vi "Spectrometer Triax 550 (N.O.).vi"(7 "Force Reset? (F)":bool, 8 "error in (no error)":errorcluster, 9 "VISA Resource Name":refnum<visa-resource-name>="GPIB0::1::INSTR", 10 "Ref to a Status Box":refnum<vi>, 11 "Cluster In":T4) -> (0 "error out":errorcluster, 3 "Cluster Out":T4)   [LabVIEW 2012]
uses:
  JY-SPEX-TRIAX/controls.llb/Monochromator System Number.ctl
  JY-SPEX-TRIAX/controls.llb/Mirror Position.ctl
  JY-SPEX-TRIAX/controls.llb/Turret Position (TRIAX).ctl
  JY-SPEX-TRIAX/JY-SPEX-TRIAX.lvlib
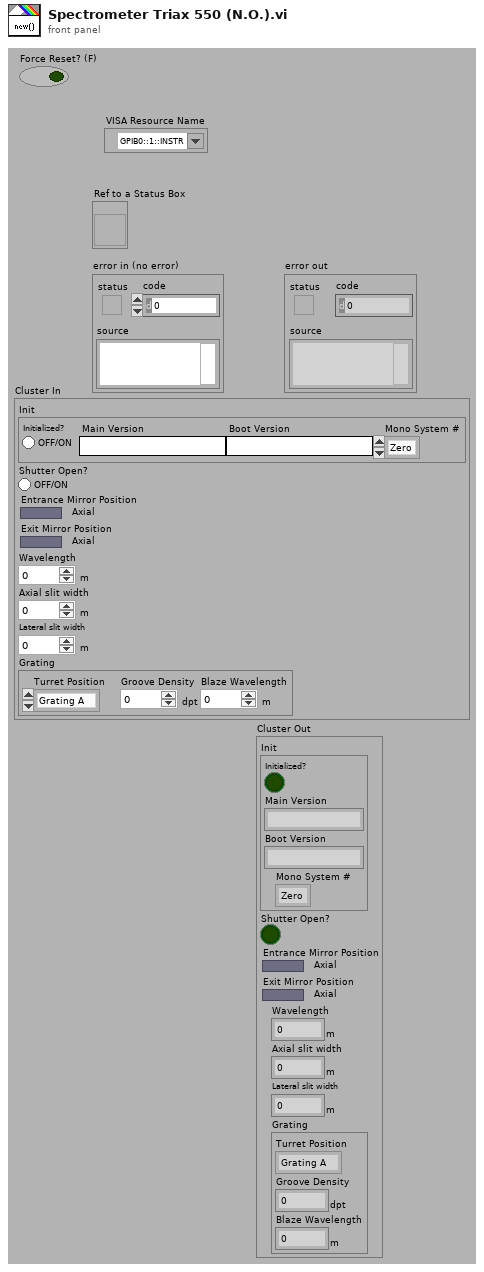
[diagram p1: front panel]
types:
  T1 = typedef "JY-SPEX-TRIAX.lvlib/Monochromator System Number.ctl" = enum16{"Zero", "One"}
  T2 = typedef "JY-SPEX-TRIAX.lvlib/Mirror Position.ctl" = bool
  T3 = typedef "JY-SPEX-TRIAX.lvlib/Turret Position (TRIAX).ctl" = enum16{"Grating A", "Grating B", "Grating C"}
  T4 = cluster{"Init":cluster{"Initialized?":bool, "Main Version":string, "Boot Version":string, "Mono System #":T1}, "Shutter Open?":bool, "Entrance Mirror Position":T2, "Exit Mirror Position":T2, "Wavelength":dbl[unit], "Axial slit width":dbl[unit], "Lateral slit width":dbl[unit], "Grating":cluster{"Turret Position":T3, "Groove Density":dbl[unit], "Blaze Wavelength":dbl[unit]}}
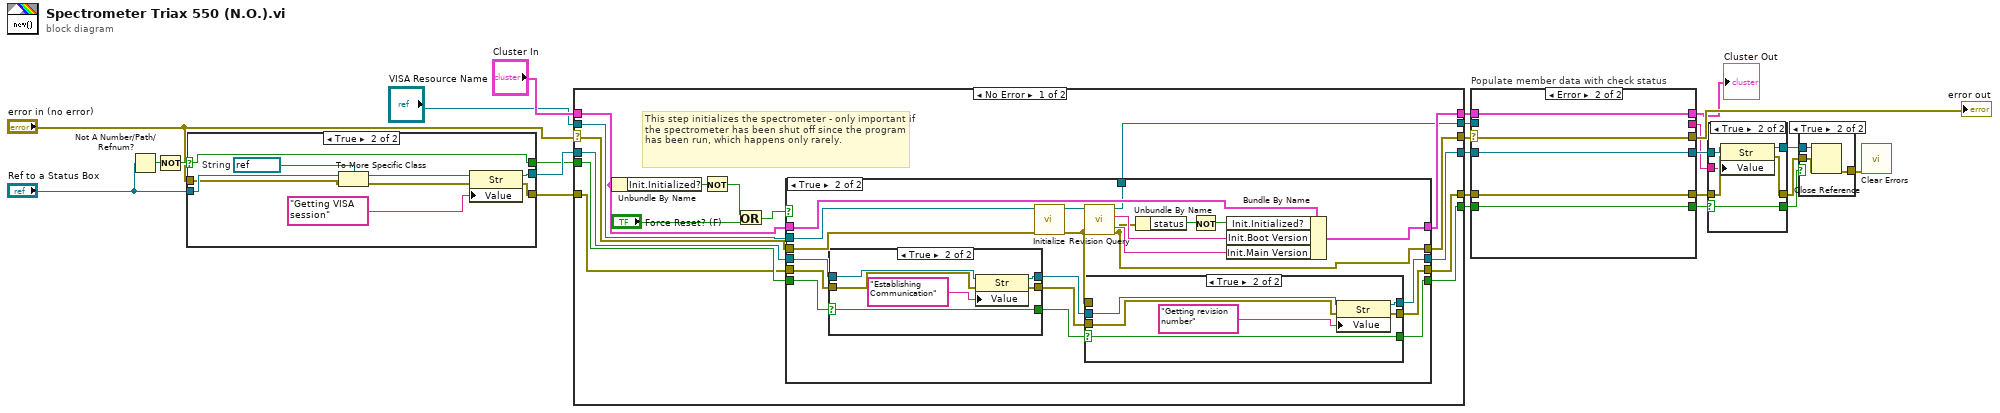
[diagram p0: block diagram]
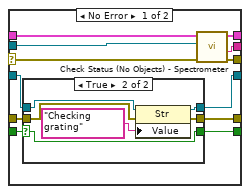
[diagram p2: hidden frame]
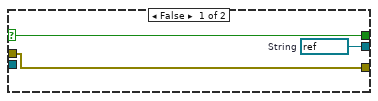
[diagram p4: hidden frame]
diagram:
  n1 = Not A Number/Path/Refnum?(number/path/refnum="Ref to a Status Box") -> (NaN/Path/Refnum?=w19:bool)
  n2 = Not(x=w19) -> (.not. x?=w7:bool)
  n3 = case shown="True" w7 {
    selector: w7 -> [w27 w34]
    tunnel: "error in (no error)" -> [w28 w29]
    tunnel: [w28 w37] -> w23
    tunnel: "Ref to a Status Box" -> [_ w32]
    tunnel: [w26 w35] -> w25
    tunnel: [w27 w34] -> w24
    frame False {
      w26 = refnum<vi> refnum  # String
    }
    frame True {
      w33 = refnum<vi> refnum  # String
      n4 = To More Specific Class(target class=w33, reference=w32, error in=w29) -> (specific class reference=w30:refnum<vi>, error out=w31:errorcluster)
      n5 = property class="Str"(reference=w30, error in=w31, "Value"="Getting VISA session") -> (reference out=w35:refnum<vi>, error out=w37:errorcluster)
    }
  }
  n6 = case shown="No Error" "error in (no error)" {
    selector: "error in (no error)" -> [w44 w104]
    tunnel: [w47 w104] -> w6
    tunnel: "Cluster In" -> [w43 w103]
    tunnel: "VISA Resource Name" -> [w53 w99]
    tunnel: [w52 w103] -> w18
    tunnel: w25 -> [w51 w102]
    tunnel: [w48 w102] -> w16
    tunnel: w24 -> [w50 w101]
    tunnel: [w49 w101] -> w14
    tunnel: w23 -> [w46 w100]
    tunnel: [w45 w100] -> w11
    tunnel: [w38 w99] -> w1
    frame No Error {
      # "This step initializes the spectrometer - only important if the spectrometer has been shut off since the program has been run, which happens only rarely."
      n7 = Unbundle By Name(w43) -> ("Init.Initialized?"=w41:bool)
      n8 = Not(x=w41) -> (.not. x?=w42:bool)
      n9 = Or(x=w42, y="Force Reset? (F)") -> (x .or. y?=w39:bool)
      n10 = case shown="True" w39 {
        tunnel: w43 -> [w59 w76]
        tunnel: w53 -> [w54 w75]
        tunnel: [w59 w62] -> w52
        tunnel: w51 -> [w57 w74]
        tunnel: w50 -> [w55 w73]
        tunnel: [w55 w71] -> w49
        tunnel: [w57 w69] -> w48
        tunnel: [w58 w61] -> w47
        tunnel: w46 -> [w56 w68]
        tunnel: [w56 w66] -> w45
        tunnel: w44 -> [w58 w65]
        tunnel: [w54 w60] -> w38
        frame False {
        }
        frame True {
          n11 = case shown="True" w73 {
            selector: w73 -> [w90 w93]
            tunnel: w68 -> [w91 w98]
            tunnel: [w91 w97] -> w67
            tunnel: w74 -> [w92 w96]
            tunnel: [w92 w94] -> w70
            tunnel: [w90 w93] -> w72
            frame False {
            }
            frame True {
              n12 = property class="Str"(reference=w96, error in=w98, "Value"="Establishing Communication") -> (reference out=w94:refnum<vi>, error out=w97:errorcluster)
            }
          }
          n13 = call "Initialize.vi"("error in (no error)"=w65, "VISA resource name"=w75) -> ("error out"=w63:errorcluster, "VISA resource name out"=w80:refnum<visa-resource-name>)  [unwired: 8 out]
          n14 = call "Revision Query.vi"("error in (no error)"=w63, "VISA resource name"=w80) -> ("error out"=w61:errorcluster, "Main Firmware Revision"=w77:string, "Boot Firmware Revision"=w78:string, "VISA resource name out"=w60:refnum<visa-resource-name>)  [unwired: 6 out]
          n15 = case shown="True" w72 {
            selector: w72 -> [w81 w84]
            tunnel: w67 -> [w82 w89]
            tunnel: [w82 w88] -> w66
            tunnel: w70 -> [w83 w87]
            tunnel: [w83 w85] -> w69
            tunnel: [w81 w84] -> w71
            tunnel: w63 -> [_ _]
            frame False {
            }
            frame True {
              n16 = property class="Str"(reference=w87, error in=w89, "Value"="Getting revision number") -> (reference out=w85:refnum<vi>, error out=w88:errorcluster)
            }
          }
          n17 = Unbundle By Name(w61) -> ("status"=w79:bool)
          n18 = Not(x=w79) -> (.not. x?=w64:bool)
          n19 = Bundle By Name(cluster=w76, "Init.Initialized?"=w64, "Init.Boot Version"=w78, "Init.Main Version"=w77) -> (w62:T4)
        }
      }
    }
    frame Error {
    }
  }
  n20 = case "Populate member data with check status" shown="Error" w6 {
    selector: w6 -> [w107 w129]
    tunnel: w18 -> [w106 w130]
    tunnel: [w116 w129] -> w17
    tunnel: [w115 w130] -> w3
    tunnel: w16 -> [w114 w127]
    tunnel: [w113 w127] -> w15
    tunnel: w14 -> [w112 w128]
    tunnel: [w111 w128] -> w13
    tunnel: [w110 w126] -> w12
    tunnel: w11 -> [w109 w126]
    tunnel: [w108 _] -> w10
    tunnel: w1 -> [w105 _]
    frame No Error {
      n21 = case shown="True" w112 {
        selector: w112 -> [w119 w123]
        tunnel: [w117 w125] -> w110
        tunnel: [w119 w123] -> w111
        tunnel: [w118 w122] -> w113
        tunnel: w109 -> [w117 w121]
        tunnel: w114 -> [w118 w120]
        frame False {
        }
        frame True {
          n22 = property class="Str"(reference=w120, error in=w121, "Value"="Checking grating") -> (reference out=w122:refnum<vi>, error out=w125:errorcluster)
        }
      }
      n23 = call "Check Status (No Objects) - Spectrometer.vi"("error in (no error)"=w107, "VISA Resource Name"=w105, "Cluster In"=w106) -> ("error out"=w116:errorcluster, "Status"=w108:string, "Cluster Out"=w115:T4)  [unwired: 5 in, 1 out]
    }
    frame Error {
    }
  }
  "error out" <- w17
  "Cluster Out" <- w3
  n24 = case shown="True" w13 {
    selector: w13 -> [w133 w137]
    tunnel: [w132 w139] -> w22
    tunnel: [w131 w138] -> w9
    tunnel: [w133 w137] -> w8
    tunnel: w15 -> [w131 w136]
    tunnel: w12 -> [w132 w135]
    tunnel: w10 -> [_ w134]
    frame False {
    }
    frame True {
      n25 = property class="Str"(reference=w136, error in=w135, "Value"=w134) -> (reference out=w138:refnum<vi>, error out=w139:errorcluster)
    }
  }
  n26 = case shown="True" w8 {
    tunnel: w22 -> [w140 w143]
    tunnel: [w140 w142] -> w21
    tunnel: w9 -> [_ w141]
    frame False {
    }
    frame True {
      n27 = Close Reference(reference=w141, error in (no error)=w143) -> (error out=w142:errorcluster)
    }
  }
  n28 = call <vilib>:"Clear Errors.vi"("error in (no error)"=w21) -> ()  [unwired: 7 out]
